vi ".vi"() -> ()   [LabVIEW 2016]
uses:
  Measure_core/Template Module/Template Module.lvclass
panel:
  out "Module":refnum<class "Template Module.lvclass">
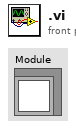
[diagram p1: front panel]
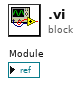
[diagram p0: block diagram]
diagram:
